vi "Microsync get property.vi"(4 "error in (no error)":errorcluster, 5 "VISA resource name":refnum<visa-resource-name>, 11 "Property":T1(ring)) -> (0 "error out":errorcluster, 2 "Property value":string, 3 "VISA resource name out":refnum<visa-resource-name>)   [LabVIEW 2023]
uses:
  aae625e4-2daa-4f28-afe9-3577fc42129b.vi
panel:
  in  "Command":string="GET"
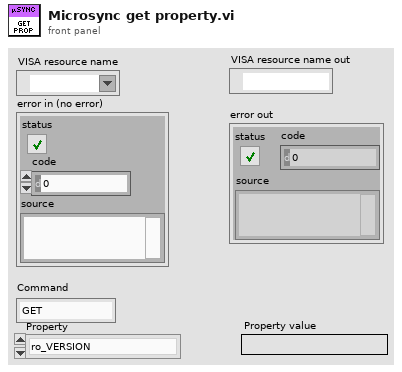
[diagram p1: front panel]
types:
  T1 = enum16{"ro_VERSION", "ro_SYS_TIMER_STATUS", "ro_SYS_TIMER_VALUE", "ro_SYS_TIMER_OVF_COUNT", "ro_SYS_TIME_ms", "ro_SYS_TIMER_PRESCALER", "rw_DFLT_PULSE_DURATION_us", "ro_WATCHDOG_TIMEOUT_ms", "ro_N_EVENTS", "rw_INTLCK_ENABLED", "rw_SELECTED_LASERS", "wo_OPEN_SHUTTERS", "wo_CLOSE_SHUTTERS", "rw_SHUTTER_DELAY_us", "rw_CAM_READOUT_us"}
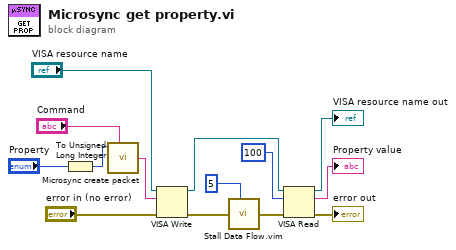
[diagram p0: block diagram]
diagram:
  n1 = To Unsigned Long Integer(number="Property") -> (unsigned 32bit integer=w9:u32)
  n2 = call "Microsync create packet.vi"("Command"="Command", "arg1"=w9) -> ("data packet"=w14:string)  [unwired: 4 in]
  n3 = VISA Write(VISA resource name="VISA resource name", write buffer=w14, error in (no error)="error in (no error)") -> (VISA resource name out=w5:refnum<visa-resource-name>, error out=w8:errorcluster)  [unwired: 1 out]
  n4 = call "Stall Data Flow.vim"("value in"=w8, "milliseconds to wait"=u32 5) -> ("value out"=w4:errorcluster)  [unwired: 1 out]
  n5 = VISA Read(VISA resource name=w5, byte count=u32 100, error in (no error)=w4) -> (VISA resource name out=→"VISA resource name out":refnum<visa-resource-name>, read buffer=→"Property value":string, error out=→"error out":errorcluster)  [unwired: 1 out]
